vi "libssh2_channel_close.vi"(8 "error in (no error)":errorcluster, 11 "Channel":T1) -> (0 "error out":errorcluster, 3 "return value":i32)   [LabVIEW 2013, in "libssh2.lvlib"]
uses:
  libssh2.lvlib
  Channel Refnum.ctl
  libssh2.dll
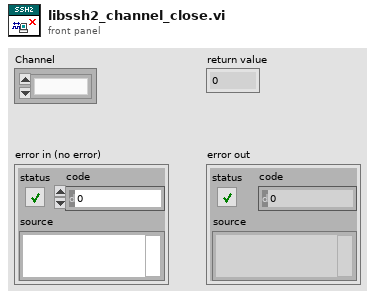
[diagram p1: front panel]
types:
  T1 = typedef "libssh2.lvlib/Channel Refnum.ctl" = refnum<k1>
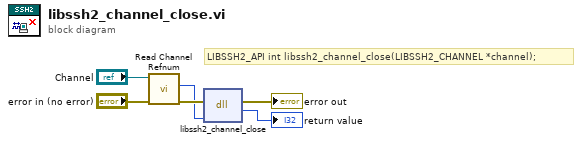
[diagram p0: block diagram]
diagram:
  # "LIBSSH2_API int libssh2_channel_close(LIBSSH2_CHANNEL *channel);"
  n1 = call "Read Channel Refnum.vi"("error in (no error)"="error in (no error)", "Channel"="Channel") -> ("error out"=w3:errorcluster, "LIBSSH2_CHANNEL*"=w2:u64)  [unwired: 8 in]
  n2 = dll-call lib="C:/Users/pasca/source/repos/libssh2-labview/libssh2**.*" fn="libssh2_channel_close"(error in=w3, "channel"=w2) -> (error out=→"error out":errorcluster, "return value"=→"return value":i32)  [unwired: 3 in, 1 out]
